vi "BasicExample.vi"() -> ()   [LabVIEW 2025]
uses:
  PalmSens/PalmSens.lvclass
  C:/Users/stef/code/palmsenssdk/labview/PalmSens/Libraries/PalmSens.Core.Simplified.LabVIEW.dll
  PalmSens/Libraries/PalmSens.Core.Simplified.LabVIEW.dll
  PalmSens/MeasurementResults.ctl
  PalmSens/LiveCurveResult.ctl
panel:
  out "Results":T1
  out "LSV Method Indicator":refnum<k24>
  out "Array":string[](array[string])
  out "Is Measuring":bool
  in  "PalmSens.lvclass":refnum<class "PalmSens.lvclass">
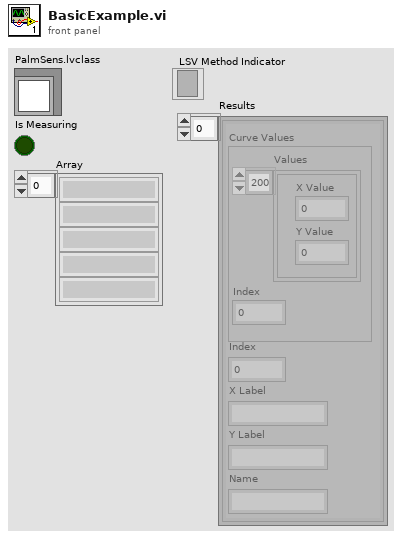
[diagram p1: front panel]
types:
  T1 = typedef "MeasurementResults.ctl" = T2[]
  T2 = typedef "LiveCurveResult.ctl" = cluster{"X Label":string, "Y Label":string, "Name":string, "Index":i16, "Curve Values":cluster{"Values":cluster{"X Value":dbl, "Y Value":dbl}[], "Index":i16}}
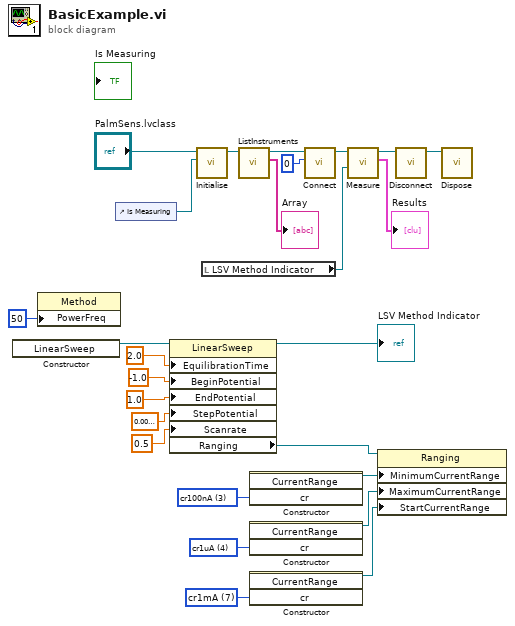
[diagram p0: block diagram]
diagram:
  w17 = 4 items=["cr100pA"=0, "cr1nA"=1, "cr10nA"=2, "cr100nA"=3, "cr1uA"=4, "cr10uA"=5, "cr100uA"=6, "cr1mA"=7, "cr10mA"=8, "cr100mA"=9, "cr2uA"=10, "cr4uA"=11, "cr8uA"=12, "cr16uA"=13, "cr32uA"=14, "cr125uA"=17, "cr250uA"=18, "cr500uA"=19, "cr5mA"=20, "cr6uA"=21, "cr13uA"=22, "cr25uA"=23, "cr50uA"=24, "cr200uA"=25, "cr63uA"=26] ("cr")
  w18 = 7 items=["cr100pA"=0, "cr1nA"=1, "cr10nA"=2, "cr100nA"=3, "cr1uA"=4, "cr10uA"=5, "cr100uA"=6, "cr1mA"=7, "cr10mA"=8, "cr100mA"=9, "cr2uA"=10, "cr4uA"=11, "cr8uA"=12, "cr16uA"=13, "cr32uA"=14, "cr125uA"=17, "cr250uA"=18, "cr500uA"=19, "cr5mA"=20, "cr6uA"=21, "cr13uA"=22, "cr25uA"=23, "cr50uA"=24, "cr200uA"=25, "cr63uA"=26] ("cr")
  w20 = 3 items=["cr100pA"=0, "cr1nA"=1, "cr10nA"=2, "cr100nA"=3, "cr1uA"=4, "cr10uA"=5, "cr100uA"=6, "cr1mA"=7, "cr10mA"=8, "cr100mA"=9, "cr2uA"=10, "cr4uA"=11, "cr8uA"=12, "cr16uA"=13, "cr32uA"=14, "cr125uA"=17, "cr250uA"=18, "cr500uA"=19, "cr5mA"=20, "cr6uA"=21, "cr13uA"=22, "cr25uA"=23, "cr50uA"=24, "cr200uA"=25, "cr63uA"=26] ("cr")
  n1 = constructor class="LinearSweep"() -> (reference out=w16:refnum<k24>)  [unwired: 3 in, 2 out]
  n2 = property class="Method"("PowerFreq"=50) -> ()  [unwired: 2 in, 2 out]
  n3 = control-ref of="Is Measuring"() -> (w25:refnum<vi>)
  n4 = property class="LinearSweep"(reference=w16, "EquilibrationTime"=sgl 2.0, "BeginPotential"=sgl -1.0, "EndPotential"=sgl 1.0, "StepPotential"=sgl 0.01, "Scanrate"=sgl 0.5) -> (reference out=→"LSV Method Indicator":refnum<k24>, "Ranging"=w3:refnum<k24>)  [unwired: 1 in, 1 out]
  n5 = call-dynamic "Initialise.vi"("Is Measuring Refnum"=w25, "PalmSens in"="PalmSens.lvclass") -> ("PalmSens out"=w24:refnum<class "PalmSens.lvclass">)  [unwired: 8 in, 1 out]
  n6 = local read "LSV Method Indicator"() -> (w8:refnum<k24>)
  n7 = call-dynamic "ListInstruments.vi"("PalmSens in"=w24) -> ("Array"=→"Array":string[], "PalmSens out"=w22:refnum<class "PalmSens.lvclass">)  [unwired: 8 in, 1 out]
  n8 = constructor class="CurrentRange"("cr"=w20) -> (reference out=w19:refnum<k24>)  [unwired: 3 in, 3 out]
  n9 = constructor class="CurrentRange"("cr"=w17) -> (reference out=w2:refnum<k24>)  [unwired: 3 in, 3 out]
  n10 = constructor class="CurrentRange"("cr"=w18) -> (reference out=w1:refnum<k24>)  [unwired: 3 in, 3 out]
  n11 = call-dynamic "Connect.vi"("Instrument Index"=0, "PalmSens in"=w22) -> ("PalmSens out"=w9:refnum<class "PalmSens.lvclass">)  [unwired: 8 in, 1 out]
  n12 = call-dynamic "Measure.vi"("Method .NET Refnum"=w8, "PalmSens in"=w9) -> ("Curves"=→"Results":T1, "PalmSens out"=w10:refnum<class "PalmSens.lvclass">)  [unwired: 2 in, 2 out]
  n13 = property class="Ranging"(reference=w3, "MinimumCurrentRange"=w19, "MaximumCurrentRange"=w2, "StartCurrentRange"=w1) -> ()  [unwired: 1 in, 2 out]
  n14 = call-dynamic "Disconnect.vi"("PalmSens in"=w10) -> ("PalmSens out"=w12:refnum<class "PalmSens.lvclass">)  [unwired: 9 in, 1 out]
  n15 = call-dynamic "Dispose.vi"("PalmSens in"=w12) -> ()  [unwired: 9 in, 2 out]
